vi "SetFirstMeasurementCycle.vi"() -> ()   [LabVIEW 2010]
panel:
  in  "FirstRoundMeasurement":bool
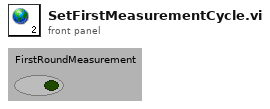
[diagram p1: front panel]
diagram:
